vi "Read_name.vi"(8 "error in (no error)":errorcluster, 11 "instrument in":refnum<class "instrument.lvclass">) -> (0 "error out":errorcluster, 2 "name":string, 3 "instrument out":refnum<class "instrument.lvclass">)   [LabVIEW 2017, in "instrument.lvclass"]
doc: "gets the name of the instrument"
uses:
  instrument.lvclass
  instrument.lvclass/instrument.ctl
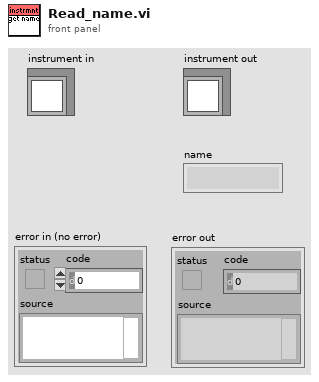
[diagram p1: front panel]
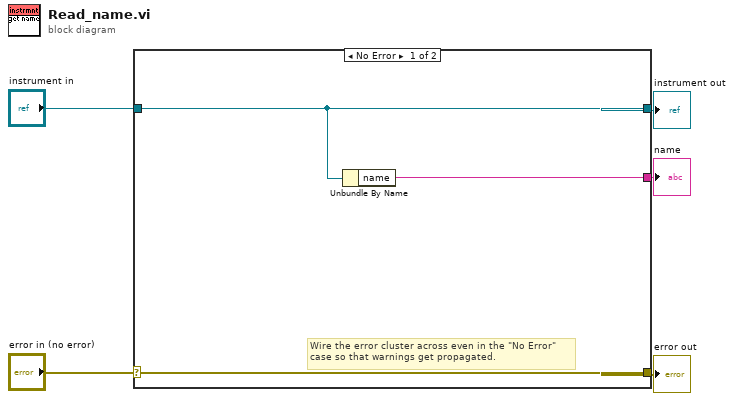
[diagram p0: block diagram]
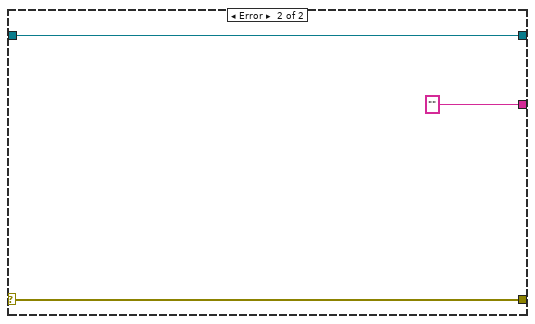
[diagram p2: hidden frame]
diagram:
  n1 = case shown="No Error" "error in (no error)" {
    selector: "error in (no error)" -> [w8 w11]
    tunnel: [w8 w11] -> w4
    tunnel: [w7 w10] -> w2
    tunnel: "instrument in" -> [w7 w10]
    tunnel: [w6 "" ("Port")] -> w1
    frame No Error {
      # "Wire the error cluster across even in the \"No Error\"\ncase so that warnings get propagated."
      n2 = Unbundle By Name(w7) -> ("name"=w6:string)
    }
    frame Error {
    }
  }
  "error out" <- w4
  "instrument out" <- w2
  "name" <- w1
